vi "Write Group Name.vi"(8 "error in (no error)":errorcluster, 10 "Group Name":string, 11 "TDMS in":refnum<class "TDMS.lvclass">) -> (0 "error out":errorcluster, 3 "TDMS out":refnum<class "TDMS.lvclass">)   [LabVIEW 2011, in "TDMS.lvclass"]
uses:
  TDMS.lvclass
  Data Type.ctl
  TDMS.lvclass/TDMS.ctl
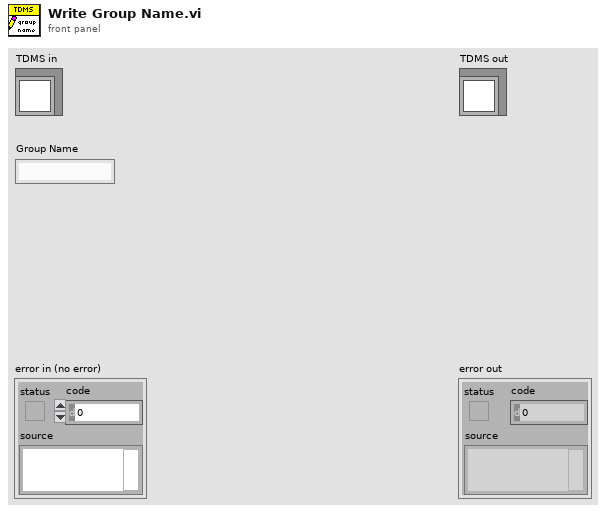
[diagram p1: front panel]
types:
  T1 = typedef "TDMS.lvclass/Data Type.ctl" = enum16{"I16", "Double", "Waveform"}
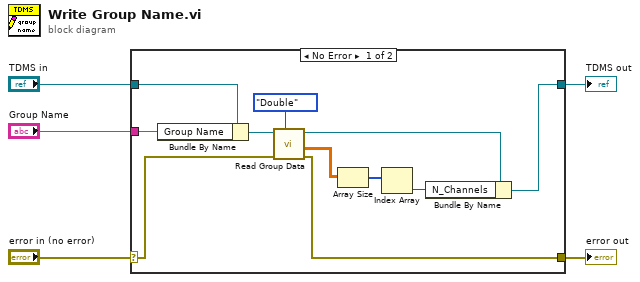
[diagram p0: block diagram]
diagram:
  n1 = case shown="No Error" "error in (no error)" {
    selector: "error in (no error)" -> [w7 w17]
    tunnel: [w6 w17] -> w4
    tunnel: [w8 w18] -> w2
    tunnel: "TDMS in" -> [w16 w18]
    tunnel: "Group Name" -> [w15 _]
    frame No Error {
      n2 = Bundle By Name(cluster=w16, "Group Name"=w15) -> (w14:refnum<class "TDMS.lvclass">)
      n3 = call "Read Group Data.vi"("data type"=Data_Type."Double", "error in"=w7, "TDMS in"=w14) -> ("error out"=w6:errorcluster, "double group data"=w11:dbl[][], "TDMS out"=w13:refnum<class "TDMS.lvclass">)  [unwired: 3 in, 3 out]
      n4 = Array Size(array=w11) -> (size(s)=w10:i32[])
      n5 = Index Array(array=w10) -> (element=w9:i32)  [unwired: 1 in]
      n6 = Bundle By Name(cluster=w13, "N_Channels"=w9) -> (w8:refnum<class "TDMS.lvclass">)
    }
    frame Error {
    }
  }
  "error out" <- w4
  "TDMS out" <- w2
